vi "Teleop.vi"(10 "Match Info":T2={"Autonomous Elapsed Seconds"=0.0, "TeleOp Elapsed Seconds"=0.0, "Disabled Elapsed Seconds"=0.0, "Visited Autonomous"=FALSE, "Visited TeleOp"=FALSE, "Visited Disabled"=FALSE, "Autonomous Settings"={"Autonomous Style"=enum."Independent", "VI Refnum"=refnum}}, 11 "Call Context":T3) -> ()   [LabVIEW 2017]
doc: "This VI is called for each TeleOp packet received from the DS where the robot is not disabled. It is often used to read from the joysticks and update I/O or to update setpoints for timed control loops. It should complete and return within 20 milliseconds or it may miss DS packets."
uses:
  <vilib>/Rock Robotics/WPI/DriverStation/WPI_DriverStationDerivedRobotMode.ctl
  <vilib>/Rock Robotics/WPI/DriverStation/WPI_DriverStationMatch Info.ctl
  <vilib>/Rock Robotics/WPI/ThirdParty/Phoenix-LabVIEW/Motor Controller/Controls/CTRE_Phoenix_MotorControl_ControlMode.ctl
  <vilib>/Rock Robotics/WPI/Utilities/WPI_GetSetVariantRefNum.vi
  <vilib>/Rock Robotics/WPI/ThirdParty/Phoenix-LabVIEW/Motor Controller/Get/CTRE_Phoenix_MotorController_GetSelectedSensorData.vi
  <vilib>/Rock Robotics/WPI/ThirdParty/Phoenix-LabVIEW/Motor Controller/Get/CTRE_Phoenix_MotorController_GetVoltage.vi
  <vilib>/Rock Robotics/WPI/ThirdParty/Phoenix-LabVIEW/Motor Controller/Get/CTRE_Phoenix_MotorController_GetOutputCurrent_Enhanced.vi
panel:
  in  "Enable Current Limit?":bool
  in  "Output":dbl
  out "Tach Velocity":dbl
  out "Mag Velocity":dbl
  out "Velocities":T1(graph)
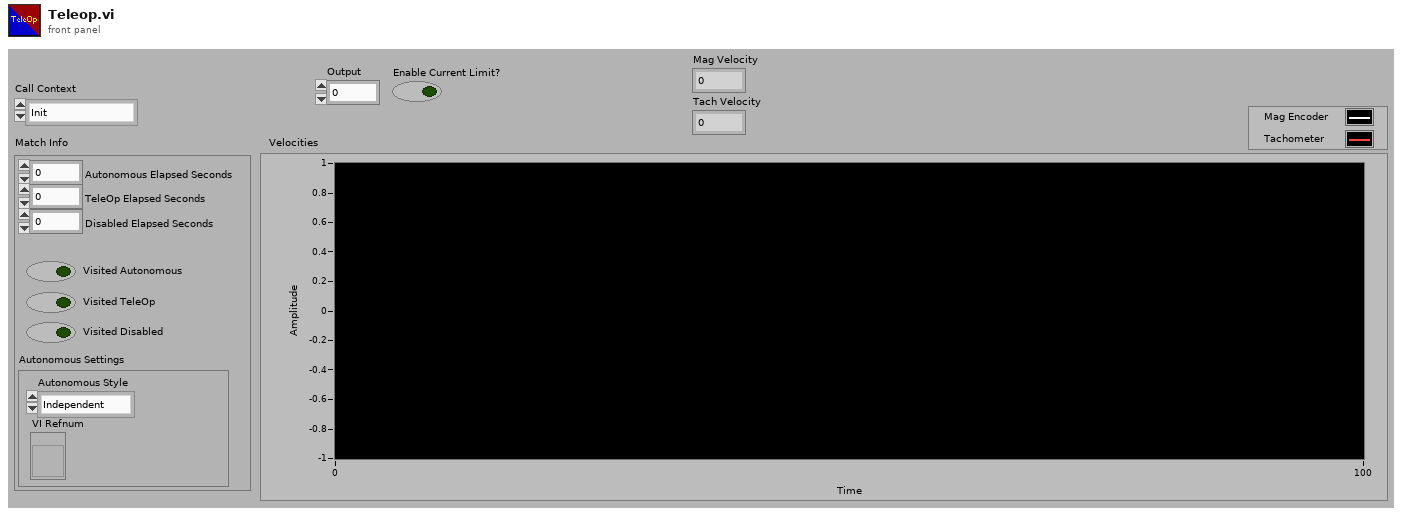
[diagram p1: front panel]
types:
  T1 = cluster{"Percent Output":dbl, "Output Current":dbl}
  T2 = typedef "WPI_DriverStationMatch Info.ctl" = cluster{"Autonomous Elapsed Seconds":dbl, "TeleOp Elapsed Seconds":dbl, "Disabled Elapsed Seconds":dbl, "Visited Autonomous":bool, "Visited TeleOp":bool, "Visited Disabled":bool, "Autonomous Settings":cluster{"Autonomous Style":enum16{"Iterative", "Independent"}, "VI Refnum":refnum<vi>}}
  T3 = typedef "WPI_DriverStationDerivedRobotMode.ctl" = enum16{"Init", "Execute", "Stop"}
  T4 = typedef "CTRE_Phoenix_MotorControl_ControlMode.ctl" = u16
  T5 = typedef "WPI_JoystickDevRef.ctl" = cluster{"Device":T6}
  T6 = typedef "WPI_JoystickDeviceEnum.ctl" = enum16{"USB 0", "USB 1", "USB 2", "USB 3", "USB 4", "USB 5"}
  T7 = typedef "WPI_MotorControlDeviceRef.ctl" = cluster{"DeviceStatus":errorcluster, "Type":T8, "PWM":cluster{"PWM Channel":T9, "DeadBand":T10}, "CAN":cluster{"Device Number":u8, "SetOutput VI Ref":variant, "GetOutput VI Ref":variant, "Enable VI Ref":variant, "Disable VI Ref":variant, "Data":variant}, "Invert":bool, "DIO PWM":cluster{"PWM \"Enable\" Channel":T9, "DIOChannel":T11, "PWM Rate":dbl}}
  T8 = typedef "WPI_MotorControlType.ctl" = enum16{"PWM", "CAN", "DIO PWM"}
  T9 = typedef "FPGA_DIOPWMChannel.ctl" = enum8{"PWM 0", "PWM 1", "PWM 2", "PWM 3", "PWM 4", "PWM 5", "PWM 6", "PWM 7", "PWM 8", "PWM 9", "PWM MXP 0", "PWM MXP 1", "PWM MXP 2", "PWM MXP 3", "PWM MXP 4", "PWM MXP 5", "PWM MXP 6", "PWM MXP 7", "PWM MXP 8", "PWM MXP 9", "Invalid"}
  T10 = typedef "WPI_PWMDeadband.ctl" = cluster{"Name":string, "maxPositivePwm":i32, "minPositivePwm":i32, "centerPwm":i32, "maxNegativePwm":i32, "minNegativePwm":i32, "angularRange":u16}
  T11 = typedef "FPGA_DIOChannel.ctl" = enum8{"DIO 0", "DIO 1", "DIO 2", "DIO 3", "DIO 4", "DIO 5", "DIO 6", "DIO 7", "DIO 8", "DIO 9", "DIO MXP 0", "DIO MXP 1", "DIO MXP 2", "DIO MXP 3", "DIO MXP 4", "DIO MXP 5", "DIO MXP 6", "DIO MXP 7", "DIO MXP 8", "DIO MXP 9", "DIO MXP 10", "DIO MXP 11", "DIO MXP 12", "DIO MXP 13", "DIO MXP 14", "DIO MXP 15", "SPI Port CS1", "SPI Port CS2", "SPI Port CS3", "SPI Port MISO", "SPI Port MOSI", "Invalid"}
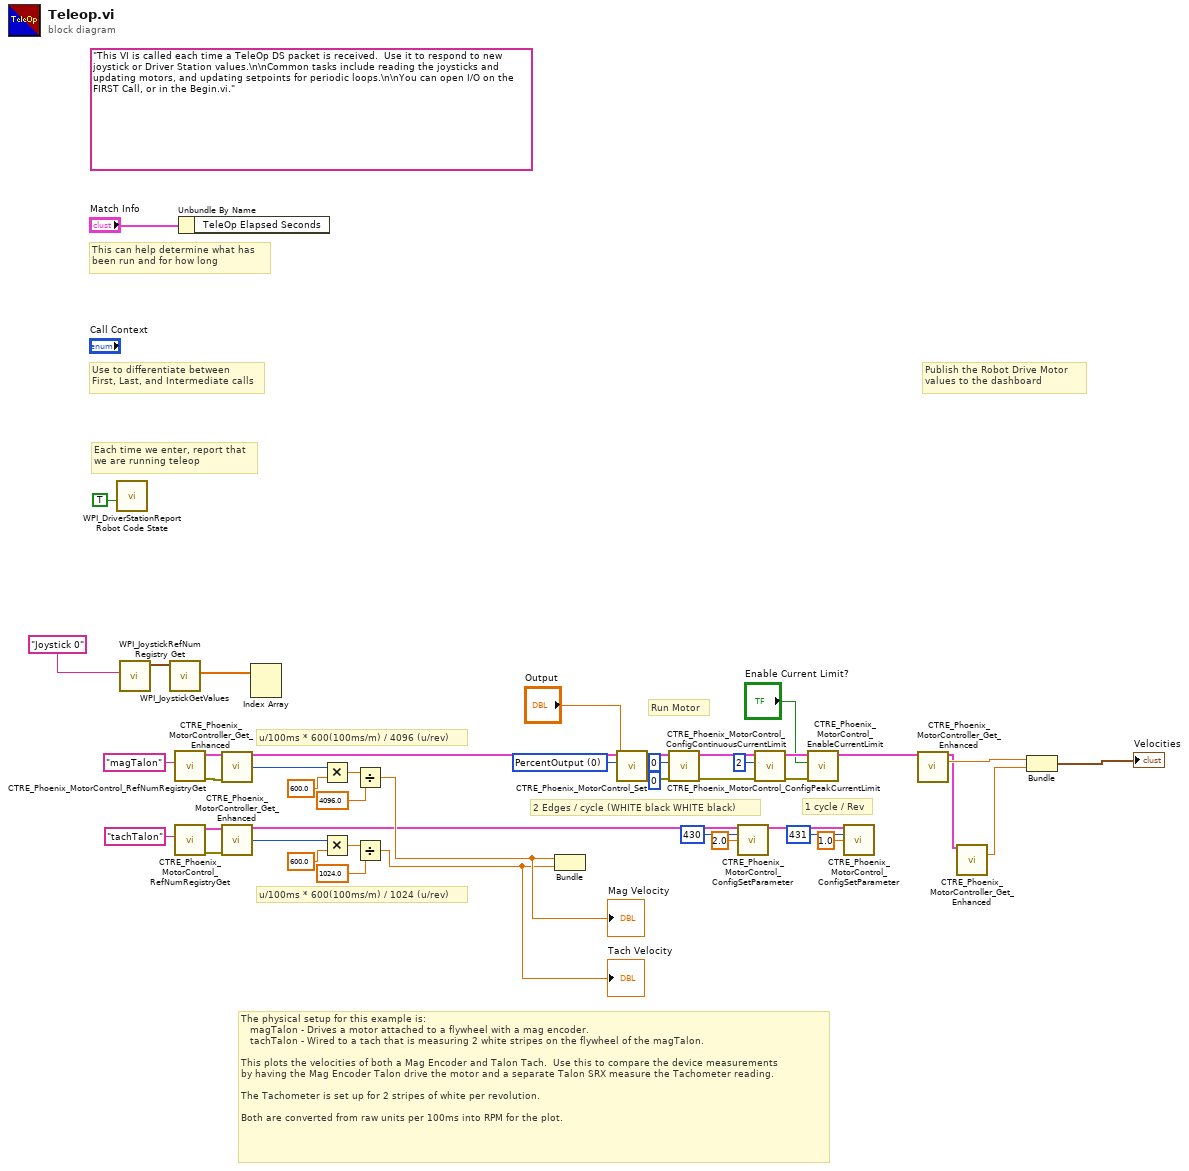
[diagram p0: block diagram]
diagram:
  w24 = T4 0 items=["PercentOutput"=0, "Position"=1, "Velocity"=2, "Current"=3, "Follower"=5, "MotionProfile"=6, "MotionMagic"=7, "MotionMagicArc"=8, "MotionProfileArc"=10, "Disabled"=15] ("Control Mode")
  (unwired) "This VI is called each time a TeleOp DS packet is received.  Use it to respond to new joystick or Driver Station values.\n\nCommon tasks include reading the joysticks and updating motors, and updating setpoints for periodic loops.\n\nYou can open I/O on the FIRST Call, or in the Begin.vi."
  # "The physical setup for this example is:\n   magTalon - Drives a motor attached to a flywheel with a mag encoder.\n   tachTalon - Wired to a tach that is measuring 2 white stripes on the flywheel of the magTalon.\n\nThis plots the velocities of both a Mag Encoder and Talon Tach.  Use this to compare the device measurements \nby having the Mag Encoder Talon drive the motor and a separate Talon SRX measure the Tachometer reading.\n\nThe Tachometer is set up for 2 stripes of white per revolution.\n\nBoth are converted from raw units per 100ms into RPM for the plot."
  # "1 cycle / Rev"
  # "2 Edges / cycle (WHITE black WHITE black)"
  # "Run Motor"
  # "u/100ms * 600(100ms/m) / 1024 (u/rev)"
  # "u/100ms * 600(100ms/m) / 4096 (u/rev)"
  # "Publish the Robot Drive Motor\nvalues to the dashboard"
  # "Each time we enter, report that\nwe are running teleop"
  # "Use to differentiate between\nFirst, Last, and Intermediate calls"
  # "This can help determine what has\nbeen run and for how long"
  n1 = call <vilib>:"WPI_DriverStationReport Robot Code State.vi"("TeleOp"=TRUE ("Autonomous")) -> ()  [unwired: 10 in, 1 out]
  n2 = call <vilib>:"WPI_JoystickRefNum Registry Get.vi"("refnum name"="Joystick 0") -> ("JoystickDevRef"=w43:T5)  [unwired: 1 in, 9 out]
  n3 = call <vilib>:"WPI_JoystickGetValues.vi"("JoystickDevRef"=w43) -> ("Axes"=w41:dbl[])  [unwired: 6 in, 4 out]
  n4 = call <vilib>:"CTRE_Phoenix_MotorControl_RefNumRegistryGet.vi"("refnum name"="magTalon") -> ("error out"=w38:errorcluster, "PhoenixMotorControlDevRef"=w37:T7)  [unwired: 9 in]
  n5 = call <vilib>:"CTRE_Phoenix_MotorControl_RefNumRegistryGet.vi"("refnum name"="tachTalon") -> ("error out"=w35:errorcluster, "PhoenixMotorControlDevRef"=w36:T7)  [unwired: 9 in]
  n6 = Unbundle By Name("Match Info") -> ()  [unwired: 1 out]
  n7 = call-poly <vilib>:"CTRE_Phoenix_MotorController_Get_Enhanced.vi"("PhoenixMotorControlDevRef"=w37, "error in"=w38) -> ("PhoenixMotorControlDevRef"=w17:T7, "Velocity (Raw Sensor Units per 100 ms)"=w31:i32)  [unwired: 10 in, 2 out]
  n8 = call-poly <vilib>:"CTRE_Phoenix_MotorController_Get_Enhanced.vi"("PhoenixMotorControlDevRef"=w36, "error in"=w35) -> ("PhoenixMotorControlDevRef"=w18:T7, "Velocity (Raw Sensor Units per 100 ms)"=w27:i32)  [unwired: 10 in, 2 out]
  n9 = Index Array(array=w41) -> ()  [unwired: 2 in, 2 out]
  n10 = Multiply(x=w31, y=600.0) -> (x*y=w34:dbl)
  n11 = Multiply(x=w27, y=600.0) -> (x*y=w28:dbl)
  n12 = Divide(x=w34, y=4096.0) -> (x/y=w26:dbl)
  "Mag Velocity" <- w26
  n13 = Divide(x=w28, y=1024.0) -> (x/y=w25:dbl)
  "Tach Velocity" <- w25
  n14 = Bundle(w26, w25) -> ()  [unwired: 1 in, 1 out]
  n15 = call <vilib>:"CTRE_Phoenix_MotorControl_Set.vi"("Output"="Output", "Control Mode"=w24, "PhoenixMotorControlDevRef"=w17) -> ("error out"=w16:errorcluster, "PhoenixMotorControlDevRef"=w15:T7)  [unwired: 7 in]
  n16 = call <vilib>:"CTRE_Phoenix_MotorControl_ConfigPeakCurrentLimit.vi"("error in (no error)"=w16, "Peak Current Maximum Duration (ms)"=0, "Peak Current (Amps)"=0, "PhoenixMotorControlDevRef"=w15) -> ("error out"=w12:errorcluster, "PhoenixMotorControlDevRef"=w11:T7)  [unwired: 6 in]
  n17 = call <vilib>:"CTRE_Phoenix_MotorControl_ConfigSetParameter.vi"("PhoenixMotorControlDevRef"=w18, "Parameter"=u32 430 ("subValue"), "value"=2.0) -> ("PhoenixMotorControlDevRef"=w19:T7)  [unwired: 11 in, 1 out]
  n18 = call <vilib>:"CTRE_Phoenix_MotorControl_ConfigContinuousCurrentLimit.vi"("error in (no error)"=w12, "Continuous Current Limit (Amps)"=2, "PhoenixMotorControlDevRef"=w11) -> ("error out"=w8:errorcluster, "PhoenixMotorControlDevRef"=w7:T7)  [unwired: 7 in]
  n19 = call <vilib>:"CTRE_Phoenix_MotorControl_EnableCurrentLimit.vi"("error in (no error)"=w8, "Enable Current Limit?"="Enable Current Limit?", "PhoenixMotorControlDevRef"=w7) -> ("PhoenixMotorControlDevRef"=w5:T7)  [unwired: 7 in, 1 out]
  n20 = call <vilib>:"CTRE_Phoenix_MotorControl_ConfigSetParameter.vi"("PhoenixMotorControlDevRef"=w19, "Parameter"=u32 431 ("subValue"), "value"=1.0) -> ()  [unwired: 11 in, 2 out]
  n21 = call-poly <vilib>:"CTRE_Phoenix_MotorController_Get_Enhanced.vi"("PhoenixMotorControlDevRef"=w5) -> ("PhoenixMotorControlDevRef"=w2:T7, "Percent Output"=w4:dbl)  [unwired: 10 in, 3 out]
  n22 = call-poly <vilib>:"CTRE_Phoenix_MotorController_Get_Enhanced.vi"("PhoenixMotorControlDevRef"=w2) -> ("Output Current"=w1:dbl)  [unwired: 12 in, 2 out]
  n23 = Bundle("Percent Output"=w4, "Output Current"=w1) -> (→"Velocities":T1)  [unwired: 1 in]
